vi "sub_PSKMod_Temp.vi"(0 "Packet to Transmit":i8[](array[numeric]), 2 "PSK system parameters":T2 {"PSK type" items=["normal", "shifted", "offset"]; "symbol map" format="%.3f"}, 7 "Symbol Rate, Hz":dbl=1.0 format="%.2f", 11 "error in (no error)":errorcluster, 12 "filter parameters":T1={"Alpha"=0.5, "Filter Length"=6, "TX Filter"=enum."Root Raised Cos"} {"Alpha" format="%.2f"}) -> (4 "output complex waveform":cluster{"t0":dbl, "dt":dbl, "Y":cdb[]} {"Y" format="%.3f"; "dt" format="%^.2e"; "t0" format="%.4f"}, 8 "samples per symbol":i32, 15 "error out":errorcluster)   [LabVIEW 2013]
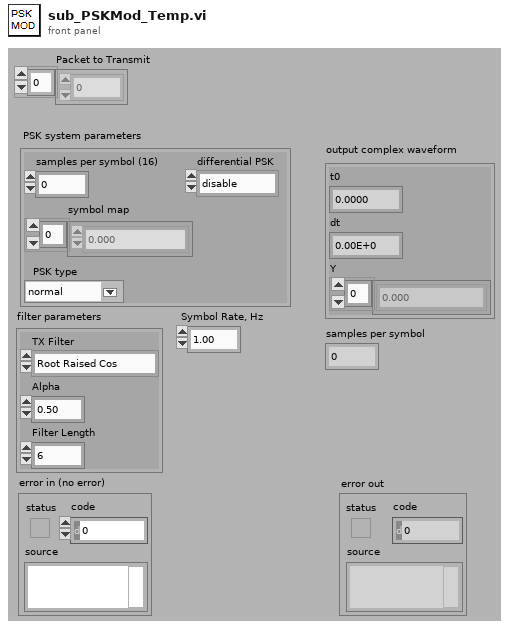
[diagram p1: front panel]
types:
  T1 = cluster{"Alpha":dbl, "Filter Length":i32, "TX Filter":enum16{"none", "Raised Cosine", "Root Raised Cos", "Gaussian"}}
  T2 = cluster{"samples per symbol (16)":i32, "symbol map":cdb[], "differential PSK":enum16{"disable", "enable"}, "PSK type":u16}
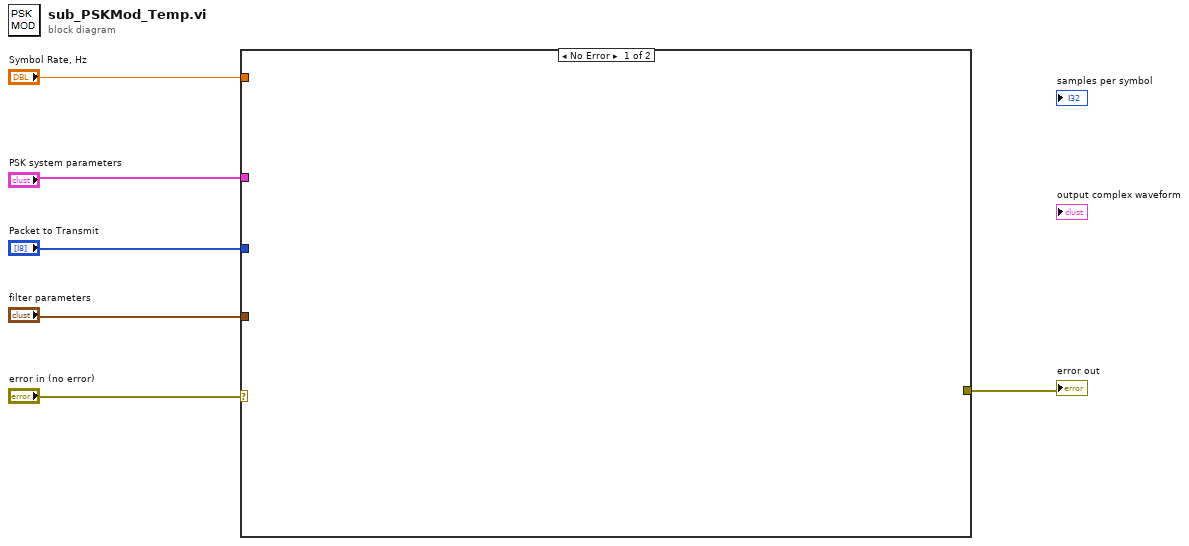
[diagram p0: block diagram]
diagram:
  n1 = case shown="No Error" "error in (no error)" {
    selector: "error in (no error)" -> [_ w7]
    tunnel: [_ w7] -> w6
    tunnel: "Symbol Rate, Hz" -> [_ _]
    tunnel: "PSK system parameters" -> [_ _]
    tunnel: "filter parameters" -> [_ _]
    tunnel: "Packet to Transmit" -> [_ _]
    frame No Error {
    }
    frame Error {
    }
  }
  "error out" <- w6
